vi "Latch.vi"(10 "clear":bool, 11 "set":bool) -> (3 "out":bool)   [LabVIEW 2021, in "Boolean_CIF_U.lvlib"]
uses:
  Boolean_CIF_U.lvlib
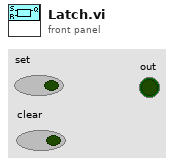
[diagram p1: front panel]
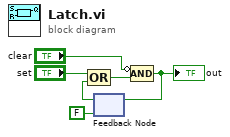
[diagram p0: block diagram]
diagram:
  n1 = feedback #1(FALSE) -> (w2:bool)
  n2 = Compound Arithmetic op=OR("set", w2) -> (w5:bool)
  n3 = Compound Arithmetic op=AND(invert "clear", w5) -> (w4:bool)
  "out" <- w4
  n4 = feedback-in #1(w4) -> ()
